vi "ep_Check dt (1 Channel).vi"(8 "error in (no error)":errorcluster, 11 "waveform in":waveform(dbl)) -> (0 "error out":errorcluster, 3 "waveform out":waveform(dbl))   [LabVIEW 2013, in "NI_EP_Power Measurement.lvlib"]
uses:
  <vilib>/addons/Electrical Power/Power Measurement/NI_EP_Power Measurement.lvlib
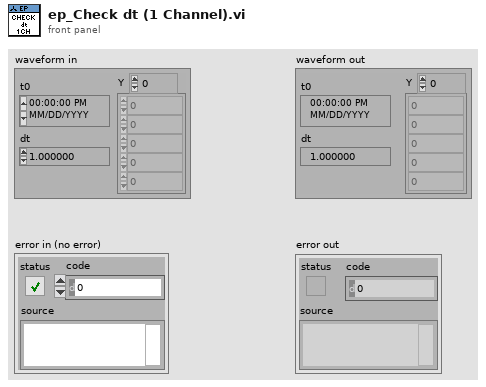
[diagram p1: front panel]
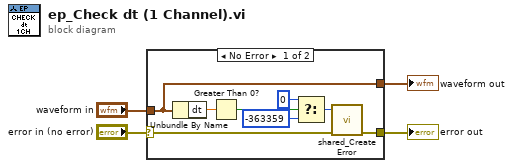
[diagram p0: block diagram]
diagram:
  n1 = case shown="No Error" "error in (no error)" {
    selector: "error in (no error)" -> [w9 w13]
    tunnel: "waveform in" -> [w5 _]
    tunnel: [w8 w13] -> w2
    tunnel: [w5 _] -> w1
    frame No Error {
      n2 = Unbundle By Name(w5) -> ("dt"=w12:dbl)
      n3 = Greater Than 0?(x=w12) -> (x > 0?=w11:bool)
      n4 = Select(t=0, s=w11, f=-363359) -> (s? t:f=w10:i32)
      n5 = call <vilib>:"shared_Create Error.vi"("error in (no error)"=w9, "error code (0)"=w10) -> ("error out"=w8:errorcluster)  [unwired: 9 in]
    }
    frame Error {
    }
  }
  "error out" <- w2
  "waveform out" <- w1
